vi "GetLastError.vi"(8 "error in (no error)":errorcluster, 11 "Status":i32) -> (0 "error out":errorcluster)   [LabVIEW 2015]
uses:
  kernel32.dll
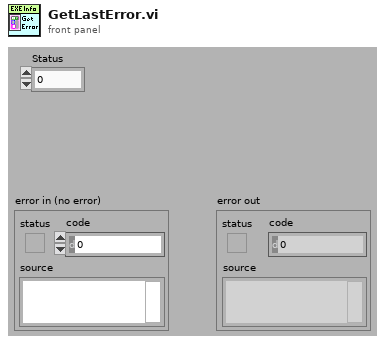
[diagram p1: front panel]
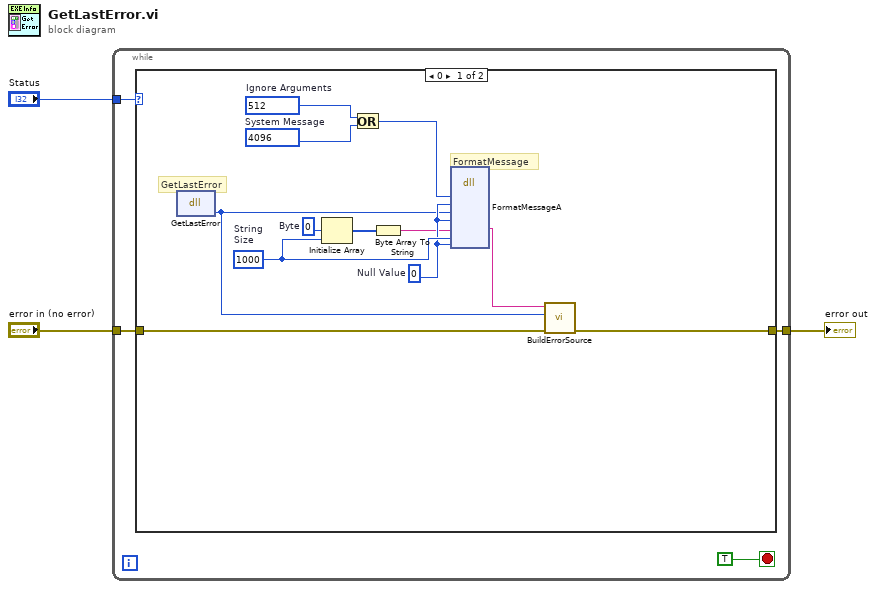
[diagram p0: block diagram]
diagram:
  n1 = while {
    tunnel: "error in (no error)" -> [w5]
    tunnel: "Status" -> [w6]
    tunnel: [w4] -> w1
    stop <- TRUE stop-if-true
    n2 = case shown="0" w6 {
      tunnel: w5 -> [w10 w20]
      tunnel: [w9 w20] -> w4
      frame 0 {
        w19 = 1000  # String Size
        w14 = u32 4096  # System Message
        w13 = u32 512  # Ignore Arguments
        w18 = u32 0  # Null Value
        w12 = u8 0  # Byte
        # "FormatMessage"
        # "GetLastError"
        n3 = dll-call lib="kernel32.dll" fn="GetLastError"() -> (w8:u32)  [unwired: 3 in, 2 out]
        n4 = Initialize Array(w12, w19) -> (w16:u8[])
        n5 = Or(x=w13, y=w14) -> (x .or. y?=w15:u32)
        n6 = Byte Array To String(unsigned byte array=w16) -> (string=w17:string)
        n7 = dll-call lib="kernel32.dll" fn="FormatMessageA"("dwFlags"=w15, "Null Value"=w18, "dwMessageId"=w8, "dwLanguageId"=w18, "lpBuffer"=w17, "nSize"=w19, "Null Value"=w18) -> ("lpBuffer"=w11:string)  [unwired: 10 in, 2 out]
        n8 = call "BuildErrorSource.vi"("error in"=w10, "status code"=w8, "extended error info"=w11) -> ("error out"=w9:errorcluster)  [unwired: 8 in]
      }
      frame 1, Default {
      }
    }
  }
  "error out" <- w1
